vi "Unhandled String Argument--error.vi"(11 "Argument":string) -> (0 "error out":errorcluster)   [LabVIEW 2020, in "MacroAssert.lvlib"]
uses:
  MacroAssert.lvlib
  <vilib>/Utility/error.llb/Error Cluster From Error Code.vi
  <vilib>/ErrorRing/Error Ring.xnode
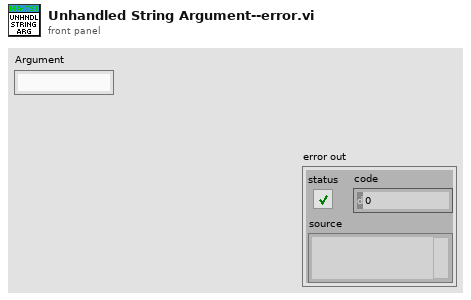
[diagram p1: front panel]
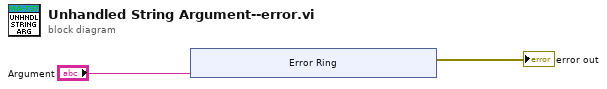
[diagram p0: block diagram]
diagram:
  n1 = xnode "Error Ring"("parameter 0"="Argument") -> ("error out"=→"error out":errorcluster)
